vi "Credit and Coin Update.vi"(8 "error in (no error)":errorcluster, 9 "Coin Value":dbl, 10 "Credit":dbl, 11 "Controller in":refnum<class "Controller.lvclass">) -> (0 "error out":errorcluster, 3 "Controller out":refnum<class "Controller.lvclass">)   [LabVIEW 2020, in "Controller.lvlib" / "Controller.lvclass"]
uses:
  Controller.lvclass
  Controller.lvclass/Controller.ctl
  Mesage Display Messages/Update Message Msg/Update Message Msg.lvclass/Update Message Msg.ctl
  <vilib>/ActorFramework/Message Enqueuer/Message Enqueuer.lvclass/Message Enqueuer.ctl
  <vilib>/ActorFramework/Message Enqueuer/Enqueue.vi
  Mesage Display Messages/Update Message Msg/Update Message Msg.lvclass
  C:/Program Files (x86)/National Instruments/LabVIEW 2020/vi.lib/ActorFramework/Message/Message.lvclass
  <vilib>/ActorFramework/Message Priority Queue/Priority Enqueue.vi
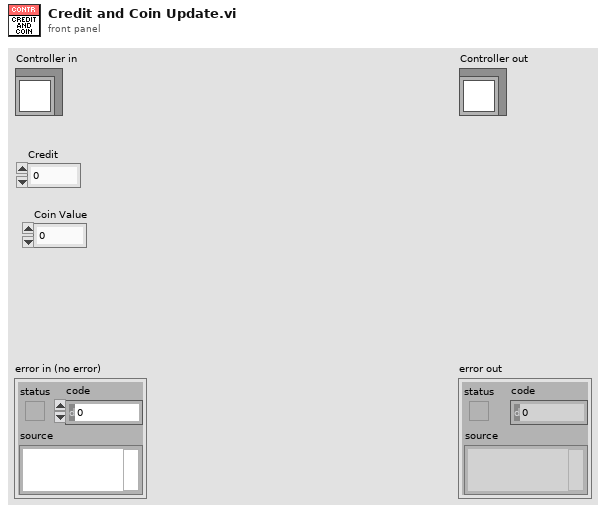
[diagram p1: front panel]
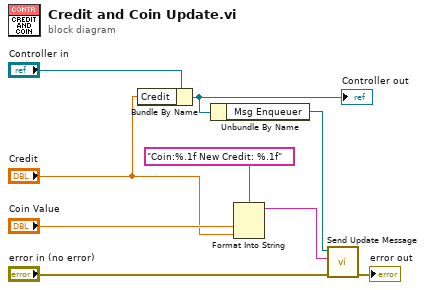
[diagram p0: block diagram]
diagram:
  n1 = Bundle By Name(cluster="Controller in", "Credit"="Credit") -> (w2:refnum<class "Controller.lvclass">)
  "Controller out" <- w2
  n2 = Unbundle By Name(w2) -> ("Msg Enqueuer"=w5:refnum<class "Message Enqueuer.lvclass">)
  n3 = Format Into String(format string="Coin:%.1f New Credit: %.1f", "Coin Value", "Credit") -> (resulting string=w7:string)  [unwired: 2 in, 1 out]
  n4 = call "Send Update Message.vi"("error in (no error)"="error in (no error)", "Msg"=w7, "Message Enqueuer"=w5) -> ("error out"=→"error out":errorcluster)  [unwired: 7 in, 1 out]
